vi "DSF.Engine.Framework.Get Status.vi"(11 "Framework in":refnum<class "DSF.Engine.Framework.lvclass">) -> (2 "Status":refnum<class "DSF.Engine.Status.Framework.lvclass">, 3 "Framework out":refnum<class "DSF.Engine.Framework.lvclass">)   [LabVIEW 2017, in "Data Sharing Framework Engine.lvlib" / "DSF.Engine.Framework.lvclass"]
uses:
  DSF.Engine.Framework.lvclass
  Status/DSF.Engine.Status.Framework.lvclass
  DSF.Engine.Framework.lvclass/DSF.Engine.Framework.ctl
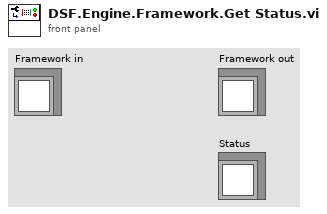
[diagram p1: front panel]
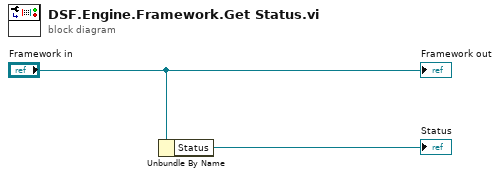
[diagram p0: block diagram]
diagram:
  n1 = Unbundle By Name("Framework in") -> ("Status"=→"Status":refnum<class "DSF.Engine.Status.Framework.lvclass">)
  "Framework out" <- "Framework in"
